vi "Get StorageLog Handle.vi"(4 "error in":errorcluster, 7 "File Path":path) -> (0 "error out":errorcluster, 1 "NaN/Path/Refnum?":bool, 3 "storage refnum (file) out":refnum<k20>)   [LabVIEW 2023]
uses:
  <vilib>/Platform/storage/lvStorage.llb/_openStorageWithRootAutoDetect.vi
  <vilib>/Platform/storage/lvStorage.llb/xStorage/xStorageSupp/ErrorOut.vi
  <vilib>/Platform/storage/lvStorage.llb/xStorage/Open Data Storage/Open Data Storage.xnode
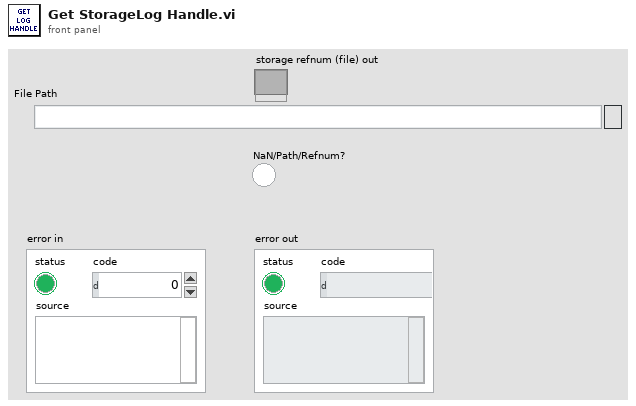
[diagram p1: front panel]
types:
  T1 = enum16{"open", "open or create", "create or replace", "create", "open (read only)"}
  T2 = enum16{"UPDATE", "READ", "QUERY", "CREATE CHILD", "CREATE", "CONNECT", "DISCONNECT"}
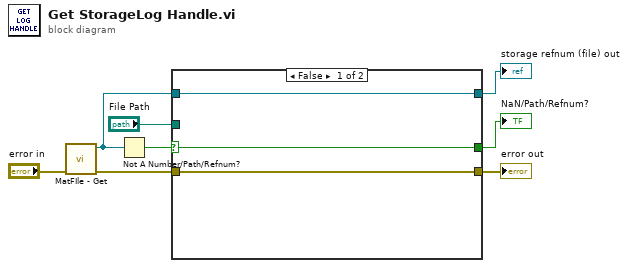
[diagram p0: block diagram]
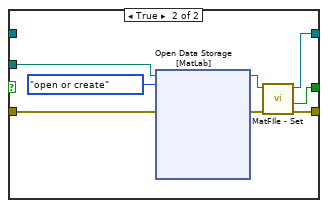
[diagram p2: hidden frame]
diagram:
  n1 = call "MatFIle - Get.vi"("error in"="error in") -> ("error out"=w6:errorcluster, "storage refnum (file) out"=w5:refnum<k20>)  [unwired: 4 in, 1 out]
  n2 = Not A Number/Path/Refnum?(number/path/refnum=w5) -> (NaN/Path/Refnum?=w8:bool)
  n3 = case shown="False" w8 {
    selector: w8 -> [w10 _]
    tunnel: "File Path" -> [_ w19]
    tunnel: w6 -> [w9 w18]
    tunnel: [w11 w14] -> w4
    tunnel: w5 -> [w11 _]
    tunnel: [w10 w13] -> w3
    tunnel: [w9 w12] -> w1
    frame False {
    }
    frame True {
      n4 = xnode "Open Data Storage\n[MatLab]"("file path"=w19, "function (open:0)"=T1."open or create", "error in (no error)"=w18) -> ("storage refnum (file)"=w16:refnum<k20>, "error out"=w15:errorcluster)  [unwired: 2 in, 1 out]
      n5 = call "MatFIle - Set.vi"("error in"=w15, "storage refnum (file) in"=w16) -> ("error out"=w12:errorcluster, "NaN/Path/Refnum?"=w13:bool, "storage refnum (file) out"=w14:refnum<k20>)  [unwired: 3 in]
    }
  }
  "NaN/Path/Refnum?" <- w3
  "storage refnum (file) out" <- w4
  "error out" <- w1
